vi "Spin to Agitate.vi"(0 "GEA2 Reference In":refnum<k24>, 1 "Standalone?":bool, 2 "Upper Limits":dbl[][](array[numeric])=[[0.0, 0.08, 4.1], [3.2, 0.08, 1.1]], 5 "GEA Inputs":T1 {"Destination" format="%.0x"; "Source" format="%.0x"}, 7 "Shift without testing?":bool, 11 "Error In":errorcluster, 13 "Lower Limits":dbl[][](array[numeric])=[[0.0, 0.02, 3.8], [2.9, 0.02, 0.7]]) -> (4 "GEA2 Reference Out":refnum<k24>, 6 "Pass/Fail?":bool, 8 "Report Text":string, 15 "Error Out":errorcluster)   [LabVIEW 2016, in "TL27.lvlib"]
uses:
  Projects/TL27.lvlib
  C:/Automation/DLLs/PC Dot Net/GeaCommunication.dll
  Common/LabVIEW GEA2 Toolkit/LabVIEW_GEA2_Toolkit.lvlibp/type defs/Source_Destination.ctl
  Common/LabVIEW GEA2 Toolkit/LabVIEW_GEA2_Toolkit.lvlibp/type defs/ERD Read Data In.ctl
  Common/LabVIEW GEA2 Toolkit/LabVIEW_GEA2_Toolkit.lvlibp/type defs/Data Type.ctl
  Common/LabVIEW GEA2 Toolkit/LabVIEW_GEA2_Toolkit.lvlibp/type defs/ERD Write Data In.ctl
  Valew Common/type defs/MC_Cycle_Engine_Request_State.ctl
  <vilib>/DAQmx/write.llb/DAQmx Write (Digital Bool 1Line 1Point).vi
  <vilib>/DAQmx/create/channels.llb/DAQmx Create Channel (DO-Digital Output).vi
  <vilib>/DAQmx/miscellaneous.llb/DAQmx Fill In Error Info.vi
  Common/LabVIEW GEA2 Toolkit/LabVIEW_GEA2_Toolkit.lvlibp
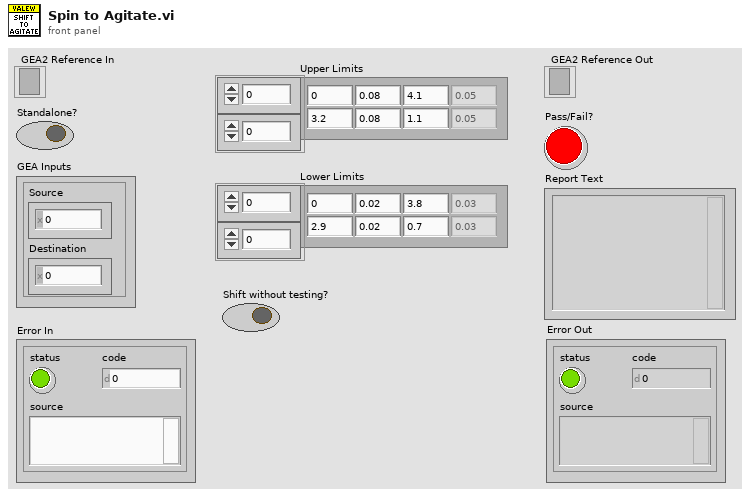
[diagram p1: front panel]
types:
  T1 = typedef "LabVIEW_GEA2_Toolkit.lvlibp/Source_Destination.ctl" = cluster{"Source":u8, "Destination":u8}
  T2 = enum16{"EQ (==)", "NE (!=)", "GT (>)", "LT (<)", "GE (>=)", "LE (<=)", "GTLT(> <)", "GELE (>= <=)", "GELT (>= <)", "GTLE (> <=)", "LTGT (< >)", "LEGE (<= >=)", "LEGT (<= >)", "LTGE (< >=)", "No Comparison"}
  T3 = typedef "LabVIEW_GEA2_Toolkit.lvlibp/ERD Read Data In.ctl" = cluster{"ERD Number":u16, "Data Type":T4}
  T4 = typedef "LabVIEW_GEA2_Toolkit.lvlibp/Data Type.ctl" = enum16{"string", "boolean", "uint8_t", "uint16_t", "uint32_t", "uint64_t", "int8_t", "int16_t", "int32_t", "int64_t"}
  T5 = typedef "LabVIEW_GEA2_Toolkit.lvlibp/ERD Write Data In.ctl" = cluster{"ERD Number":u16, "Data Type":T4, "Data":string}
  T6 = typedef "LabVIEW_GEA2_Toolkit.lvlibp/ERD Read Data Out.ctl" = cluster{"ERD Number":u16, "Data":string}
  T7 = typedef "TL27.lvlib/MC_Cycle_Engine_Request_State.ctl" = enum16{"Select", "Start", "Pause", "Resume", "Stop"}
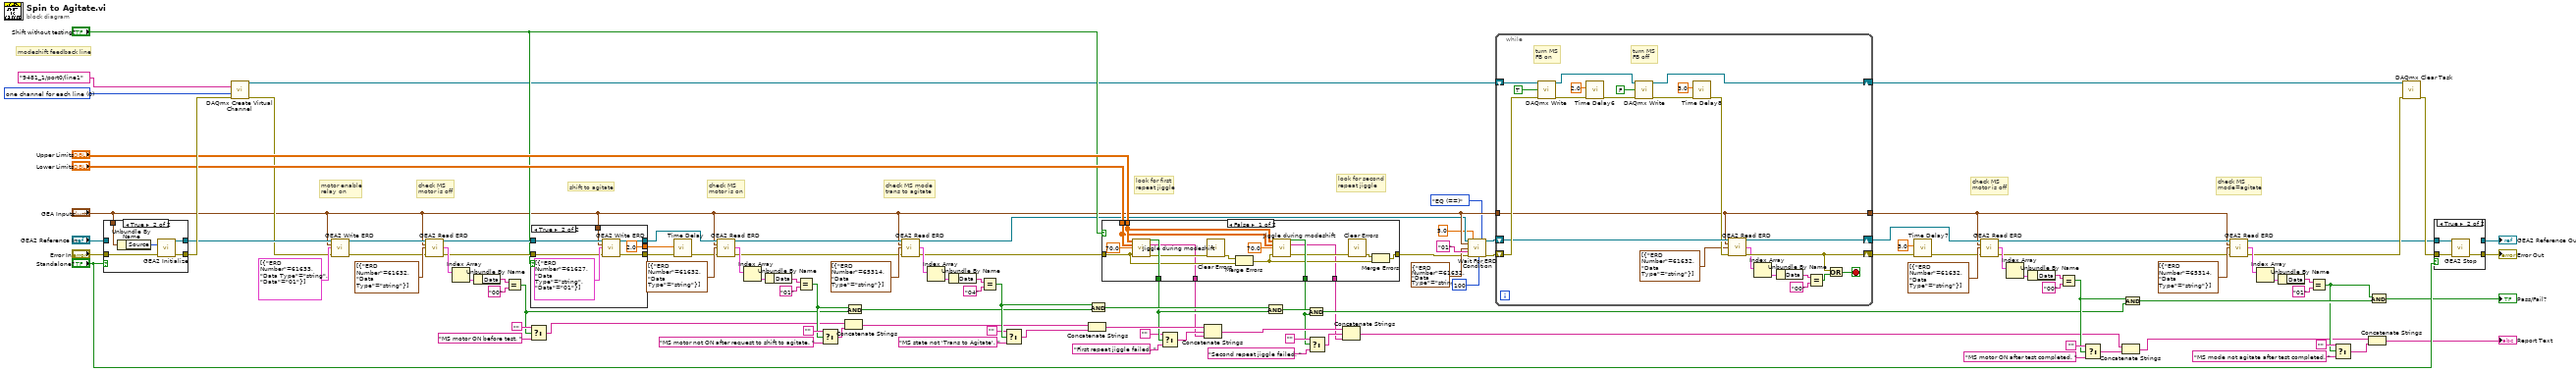
[diagram p0: block diagram]
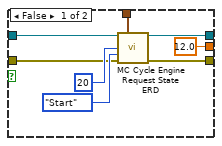
[diagram p2: hidden frame]
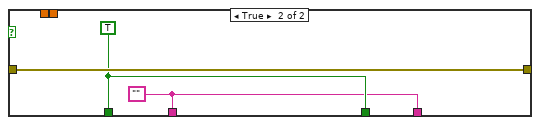
[diagram p3: hidden frame]
diagram:
  w113 = 0 items=["one channel for each line", "one channel for all lines"] ("line grouping")
  # "shift to agitate"
  # "modeshift feedback line"
  # "look for second\nrepeat jiggle"
  # "look for first\nrepeat jiggle"
  # "check MS\nmode=agitate"
  # "check MS\nmotor is off"
  # "check MS mode\ntrans to agitate"
  # "check MS\nmotor is on"
  # "check MS\nmotor is off"
  # "motor enable\nrelay on"
  n1 = case shown="True" "Standalone?" {
    tunnel: [w115 w121] -> w16
    tunnel: "Error In" -> [w116 w117]
    tunnel: [w116 w120] -> w64
    tunnel: "GEA2 Reference In" -> [w115 _]
    tunnel: "GEA Inputs" -> [_ w119]
    frame False {
    }
    frame True {
      n2 = Unbundle By Name(w119) -> ("Source"=w118:u8)
      n3 = call "GEA2 Initialize.vi"("Source Address"=w118, "error in"=w117) -> ("GEA2 Reference Out"=w121:refnum<k24>, "error out"=w120:errorcluster)  [unwired: 11 in, 1 out]
    }
  }
  n4 = call-poly <vilib>:"DAQmx Create Virtual Channel.vi"("lines"=tag "9481_1/port0/line1", "line grouping"=w113, "error in"=w64) -> ("task out"=w17:refnum<k21>, "error out"=w15:errorcluster)  [unwired: 11 in]
  n5 = call "GEA2 Write ERD.vi"("GEA2 Reference In"=w16, "GEA Inputs"="GEA Inputs", "Write ERD List"=T5[] [{"ERD Number"=61633, "Data Type"=enum."string", "Data"="01"}], "Error In"=w15) -> ("GEA2 Reference Out"=w105:refnum<k24>, "Error Out"=w104:errorcluster)  [unwired: 9 in, 1 out]
  n6 = call "GEA2 Read ERD.vi"("GEA2 Reference In"=w105, "GEA Inputs"="GEA Inputs", "Read ERD List"=T3[] [{"ERD Number"=61632, "Data Type"=enum."string"}], "Error In"=w104) -> ("GEA2 Reference Out"=w98:refnum<k24>, "ERD Data Out"=w109:T6[], "Error Out"=w97:errorcluster)  [unwired: 8 in, 1 out]
  n7 = Index Array(array=w109) -> (element=w108:T6)  [unwired: 1 in]
  n8 = Unbundle By Name(w108) -> ("Data"=w106:string)
  n9 = Equal?(x=w106, y="00") -> (x = y?=w87:bool)
  n10 = Select(t="", s=w87, f="MS motor ON before test. " ("y")) -> (s? t:f=w86:string)
  n11 = case shown="True" "Shift without testing?" {
    tunnel: w98 -> [w126 w135]
    tunnel: w97 -> [w123 w134]
    tunnel: [w125 w133] -> w89
    tunnel: [w124 w132] -> w72
    tunnel: "GEA Inputs" -> [w127 w131]
    tunnel: [12.0 ("Delay Time (s)") 2.0 ("Delay Time (s)")] -> w23
    frame False {
      n12 = call "MC Cycle Engine Request State ERD.vi"("GEA2 Reference In"=w126, "GEA Inputs"=w127, "Cycle #"=u8 20, "MC Cycle Engine State"=MC_Cycle_Engine_Request_State."Start", "Error In"=w123) -> ("GEA2 Reference Out"=w125:refnum<k24>, "Error Out"=w124:errorcluster)  [unwired: 9 in]
    }
    frame True {
      n13 = call "GEA2 Write ERD.vi"("GEA2 Reference In"=w135, "GEA Inputs"=w131, "Write ERD List"=T5[] [{"ERD Number"=61627, "Data Type"=enum."string", "Data"="01"}], "Error In"=w134) -> ("GEA2 Reference Out"=w133:refnum<k24>, "Error Out"=w132:errorcluster)  [unwired: 9 in, 1 out]
    }
  }
  n14 = call "Time Delay"("error in (no error)"=w72, "Delay Time (s)"=w23) -> ("error out"=w71:errorcluster)  [unwired: 9 in]
  n15 = call "GEA2 Read ERD.vi"("GEA2 Reference In"=w89, "GEA Inputs"="GEA Inputs", "Read ERD List"=T3[] [{"ERD Number"=61632, "Data Type"=enum."string"}], "Error In"=w71) -> ("GEA2 Reference Out"=w75:refnum<k24>, "ERD Data Out"=w96:T6[], "Error Out"=w73:errorcluster)  [unwired: 8 in, 1 out]
  n16 = Index Array(array=w96) -> (element=w95:T6)  [unwired: 1 in]
  n17 = Unbundle By Name(w95) -> ("Data"=w93:string)
  n18 = Equal?(x=w93, y="01") -> (x = y?=w88:bool)
  n19 = Select(t="", s=w88, f="MS motor not ON after request to shift to agitate. " ("y")) -> (s? t:f=w85:string)
  n20 = Concatenate Strings(w86, w85) -> (w74:string)
  n21 = And(x=w88, y=w87) -> (x .and. y?=w69:bool)
  n22 = call "GEA2 Read ERD.vi"("GEA2 Reference In"=w75, "GEA Inputs"="GEA Inputs", "Read ERD List"=T3[] [{"ERD Number"=65314, "Data Type"=enum."string"}], "Error In"=w73) -> ("GEA2 Reference Out"=w9:refnum<k24>, "ERD Data Out"=w76:T6[], "Error Out"=w70:errorcluster)  [unwired: 8 in, 1 out]
  n23 = Index Array(array=w76) -> (element=w77:T6)  [unwired: 1 in]
  n24 = Unbundle By Name(w77) -> ("Data"=w79:string)
  n25 = Equal?(x=w79, y="04") -> (x = y?=w83:bool)
  n26 = Select(t="", s=w83, f="MS state not 'Trans to Agitate'. " ("y")) -> (s? t:f=w84:string)
  n27 = Concatenate Strings(w74, w84) -> (w67:string)
  n28 = And(x=w83, y=w69) -> (x .and. y?=w68:bool)
  n29 = case shown="False" "Shift without testing?" {
    tunnel: w70 -> [w144 w154]
    tunnel: [w141 w154] -> w7
    tunnel: "Upper Limits" -> [w149 _]
    tunnel: "Lower Limits" -> [w148 _]
    tunnel: [w147 w153] -> w30
    tunnel: [w146 w153] -> w24
    tunnel: [w138 w152] -> w2
    tunnel: [w137 w152] -> w1
    frame False {
      n30 = call "Jiggle during modeshift.vi"("Upper Limits"=w149, "Lower Limits"=w148, "Timeout (s)"=70.0, "Error In"=w144) -> ("Pass/Fail?"=w147:bool, "Report Text"=w138:string, "Error Out"=w145:errorcluster)  [unwired: 8 in, 1 out]
      n31 = call <vilib>:"Clear Errors.vi"("error in (no error)"=w145) -> ("error out"=w143:errorcluster)  [unwired: 5 in, 1 out]
      n32 = Merge Errors(w143, w144) -> (w139:errorcluster)
      n33 = call "Jiggle during modeshift.vi"("Upper Limits"=w149, "Lower Limits"=w148, "Timeout (s)"=70.0, "Error In"=w139) -> ("Pass/Fail?"=w146:bool, "Report Text"=w137:string, "Error Out"=w142:errorcluster)  [unwired: 8 in, 1 out]
      n34 = call <vilib>:"Clear Errors.vi"("error in (no error)"=w142) -> ("error out"=w140:errorcluster)  [unwired: 5 in, 1 out]
      n35 = Merge Errors(w140, w139) -> (w141:errorcluster)
    }
    frame True {
      w152 = ""
      w153 = TRUE ("Pass/Fail?")
    }
  }
  n36 = Select(t="", s=w30, f="First repeat jiggle failed. " ("y")) -> (s? t:f=w31:string)
  n37 = Concatenate Strings(w67, w31, w2) -> (w65:string)
  n38 = And(x=w68, y=w30) -> (x .and. y?=w66:bool)
  n39 = And(x=w66, y=w24) -> (x .and. y?=w20:bool)
  n40 = Select(t="", s=w24, f="Second repeat jiggle failed. " ("y")) -> (s? t:f=w26:string)
  n41 = Concatenate Strings(w65, w26, w1) -> (w21:string)
  n42 = call "Wait For ERD Condition.vi"("GEA2 Reference In"=w9, "GEA Inputs"="GEA Inputs", "ERD Read Data"=T3 {"ERD Number"=61632, "Data Type"=enum."string"} ("ERD Read Data In"), "Expected Low"="01", "Error In"=w7, "Timeout (s)"=5.0, "Loop Rate (ms)"=u32 100, "Comparison"=T2."EQ (==)") -> ("GEA2 Reference Out"=w6:refnum<k24>, "Error Out"=w12:errorcluster)  [unwired: 7 in, 3 out]
  n43 = while {
    shift-right: [w159] -> w18
    shift-left: w12 -> [w162]
    shift-right: [w167] -> w14
    shift-left: w17 -> [w168]
    shift-right: [w155] -> w19
    shift-left: w6 -> [w161]
    tunnel: "GEA Inputs" -> [w158]
    tunnel: [w158] -> w13
    stop <- w164 stop-if-true
    # "turn MS\nFB on"
    # "turn MS\nFB off"
    n44 = call-poly <vilib>:"DAQmx Write.vi"("task/channels in"=w168, "data"=TRUE, "error in"=w162) -> ("task out"=w170:refnum<k21>, "error out"=w171:errorcluster)  [unwired: 10 in, 1 out]
    n45 = call "Time Delay6"("error in (no error)"=w171, "Delay Time (s)"=2.0) -> ("error out"=w169:errorcluster)  [unwired: 9 in]
    n46 = call-poly <vilib>:"DAQmx Write.vi"("task/channels in"=w170, "data"=FALSE, "error in"=w169) -> ("task out"=w167:refnum<k21>, "error out"=w165:errorcluster)  [unwired: 10 in, 1 out]
    n47 = call "Time Delay8"("error in (no error)"=w165, "Delay Time (s)"=3.0) -> ("error out"=w160:errorcluster)  [unwired: 9 in]
    n48 = call "GEA2 Read ERD.vi"("GEA2 Reference In"=w161, "GEA Inputs"=w158, "Read ERD List"=T3[] [{"ERD Number"=61632, "Data Type"=enum."string"}], "Error In"=w160) -> ("GEA2 Reference Out"=w155:refnum<k24>, "ERD Data Out"=w156:T6[], "Error Out"=w159:errorcluster)  [unwired: 8 in, 1 out]
    n49 = Index Array(array=w156) -> (element=w177:T6)  [unwired: 1 in]
    n50 = Unbundle By Name(w177) -> ("Data"=w176:string)
    n51 = Equal?(x=w176, y="00") -> (x = y?=w163:bool)
    n52 = Or(x=w159, y=w163) -> (x .or. y?=w164:bool)
  }
  n53 = call "Time Delay7"("error in (no error)"=w18, "Delay Time (s)"=3.0) -> ("error out"=w32:errorcluster)  [unwired: 9 in]
  n54 = call "GEA2 Read ERD.vi"("GEA2 Reference In"=w19, "GEA Inputs"=w13, "Read ERD List"=T3[] [{"ERD Number"=61632, "Data Type"=enum."string"}], "Error In"=w32) -> ("GEA2 Reference Out"=w46:refnum<k24>, "ERD Data Out"=w63:T6[], "Error Out"=w47:errorcluster)  [unwired: 8 in, 1 out]
  n55 = Index Array(array=w63) -> (element=w62:T6)  [unwired: 1 in]
  n56 = Unbundle By Name(w62) -> ("Data"=w60:string)
  n57 = Equal?(x=w60, y="00") -> (x = y?=w55:bool)
  n58 = Select(t="", s=w55, f="MS motor ON after test completed. " ("y")) -> (s? t:f=w56:string)
  n59 = Concatenate Strings(w21, w56) -> (w43:string)
  n60 = And(x=w55, y=w20) -> (x .and. y?=w45:bool)
  n61 = call "GEA2 Read ERD.vi"("GEA2 Reference In"=w46, "GEA Inputs"=w13, "Read ERD List"=T3[] [{"ERD Number"=65314, "Data Type"=enum."string"}], "Error In"=w47) -> ("GEA2 Reference Out"=w39:refnum<k24>, "ERD Data Out"=w54:T6[], "Error Out"=w41:errorcluster)  [unwired: 8 in, 1 out]
  n62 = Index Array(array=w54) -> (element=w53:T6)  [unwired: 1 in]
  n63 = Unbundle By Name(w53) -> ("Data"=w51:string)
  n64 = Equal?(x=w51, y="01") -> (x = y?=w44:bool)
  n65 = Select(t="", s=w44, f="MS mode not agitate after test completed. " ("y")) -> (s? t:f=w42:string)
  n66 = Concatenate Strings(w43, w42) -> (→"Report Text":string)
  n67 = And(x=w44, y=w45) -> (x .and. y?=→"Pass/Fail?":bool)
  n68 = call <vilib>:"DAQmx Clear Task.vi"("task in"=w14, "error in"=w41) -> ("error out"=w40:errorcluster)  [unwired: 13 in]
  n69 = case shown="True" "Standalone?" {
    tunnel: w39 -> [w179 w182]
    tunnel: w40 -> [w178 w181]
    tunnel: [w179 _] -> w110
    tunnel: [w178 w180] -> w38
    frame False {
    }
    frame True {
      n70 = call "GEA2 Stop.vi"("GEA2 Reference In"=w182, "Error In"=w181) -> ("Error Out"=w180:errorcluster)  [unwired: 13 in]
    }
  }
  "GEA2 Reference Out" <- w110
  "Error Out" <- w38
